vi "countArrAvgSum.vi"(1 "Array 2":dbl[](array[numeric])) -> (0 "VidejaVertiba":dbl)   [LabVIEW 2025]
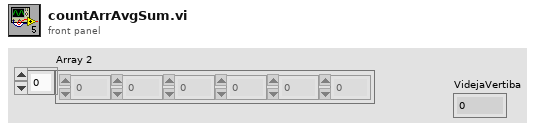
[diagram p1: front panel]
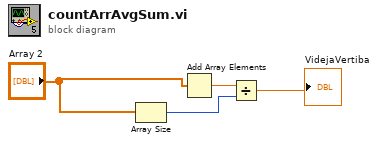
[diagram p0: block diagram]
diagram:
  n1 = Array Size(array="Array 2") -> (size(s)=w4:i32)
  n2 = Add Array Elements(numeric array="Array 2") -> (sum=w2:dbl)
  n3 = Divide(x=w2, y=w4) -> (x/y=→"VidejaVertiba":dbl)
